vi "trial code new pid.vi"() -> ()   [LabVIEW 2025]
uses:
  <vilib>/Instr/_visa.llb/VISA Configure Serial Port (Instr).vi
  <vilib>/addons/control/pid/NI_PID_pid.lvlib
  <vilib>/addons/control/pid/pid.llb/PID (DBL).vi
  <vilib>/numeric/Random Number (Range) DBL.vi
panel:
  in  "lower bound (0)":dbl
  in  "Stroke 2":dbl
  out "error out":errorcluster
  out "Stroke RAW":dbl
  out "Stroke Tare":dbl
  in  "Boolean":bool
  in  "PID SEND":bool
  in  "PID ON":bool
  in  "Stop 3":bool
  out "output Vpp":dbl
  in  "input variable":dbl=1.0
  in  "Stop 2":bool
  out "Stroke":dbl
  out "cof":dbl
  out "Friction":dbl
  out "pizo raw":dbl
  out "LVDT Peak":dbl
  out "LVDT MAX":dbl
  out "LVDT MIN":dbl
  in  "Stroke PID Gains 2":T1={"Proportional Gain (Kc)"=200.0, "Integral Time (Ti, min)"=0.02, "Derivative Time (Td, min)"=0.0}
  in  "STROKE GAIN :":dbl=700.0 caption="Stroke Gain :"
  in  "Set Strk":dbl=1.0 caption="STROKE LENGTH" min=1.0 max=1.0 step=1.0 format="%.3f"
  in  "PID Rst":bool=TRUE
  out "Stroke PID OUT":dbl(slide)=-13.483146067415703 scale=-600.0..600.0
  out "stop cmd":bool
  out "st gain":string="0000"
  out "PID Out":u8(slide) scale=0.0..4095.0
  out "start en":bool=TRUE
  in  "command":string
  in  "Stop":bool
  in  "Com Port 2":refnum<visa-resource-name>="COM9" caption="C2 :"
  out "Residual Uno 2":string
  out "Port 1 Error 2":errorcluster={"status"=TRUE, "code"=-1073807343, "source"="Property Node (arg 1) in VISA Configure Serial Port (Instr).vi->Winducom 2010--std ed hfrr-wo1768-V18.vi"}
  out "Uno Stroke":string
  out "Sps 4":dbl
  out "Port 1a 2":bool caption="Port 1 a"
  out "Port 2":u32(graph)
  out "Error Uno 2":errorcluster={"status"=TRUE, "code"=-1073807343, "source"="Property Node (arg 1) in VISA Configure Serial Port (Instr).vi->Winducom 2010--std ed hfrr-wo1768-V18.vi"}
  out "Port 4":bool=TRUE caption="Port 1"
  in  "Re-initialize Port1 2":bool
  out "Residual Uno":string
  out "Port 1 Error":errorcluster={"status"=TRUE, "code"=-1073807343, "source"="Property Node (arg 1) in VISA Configure Serial Port (Instr).vi->Winducom 2010--std ed hfrr-wo1768-V18.vi"}
  out "due":string
  out "Sps 3":dbl
  out "Port 1a":bool caption="Port 1 a"
  out "Port 1":u32(graph)
  out "Error Uno":errorcluster={"status"=TRUE, "code"=-1073807343, "source"="Property Node (arg 1) in VISA Configure Serial Port (Instr).vi->Winducom 2010--std ed hfrr-wo1768-V18.vi"}
  out "Port 3":bool=TRUE caption="Port 1"
  in  "Re-initialize Port1":bool
  out "FF buffer":dbl[](graph)
  in  "Com Port 1":refnum<visa-resource-name>="COM7" caption="C1 :"
  out "Test \nStatus":bool caption="Test Status"
types:
  T1 = cluster{"Proportional Gain (Kc)":dbl, "Integral Time (Ti, min)":dbl, "Derivative Time (Td, min)":dbl}
  T2 = cluster{"Read Heave and Surge":string, "Bytes at Heave Port":dbl, "Heave and Surge COM Port:":refnum<visa-resource-name>, "Com Port 2":refnum<visa-resource-name>, "Residual Due":string, "Heave COM Status 2":bool, "Heave COM Status":bool, "Port 2":bool, "Sway PPR":dbl, "Surge PPR":dbl, "Heave PPR":dbl, "Sway Pitch":dbl, "Surge Pitch":dbl, "Heave Pitch":dbl, "Sway Pulses/mm":dbl, "Surge Pulses/mm":dbl, "Heave Pulses/mm":dbl, "inner loop":dbl, "Read Heave and Surge 2":string, "String 36":string, "Write S":bool, "WriteCC1":string[], "Heave COM Loop":i32, "LastCom":string, "EXIT":bool, "Error Heave":errorcluster}
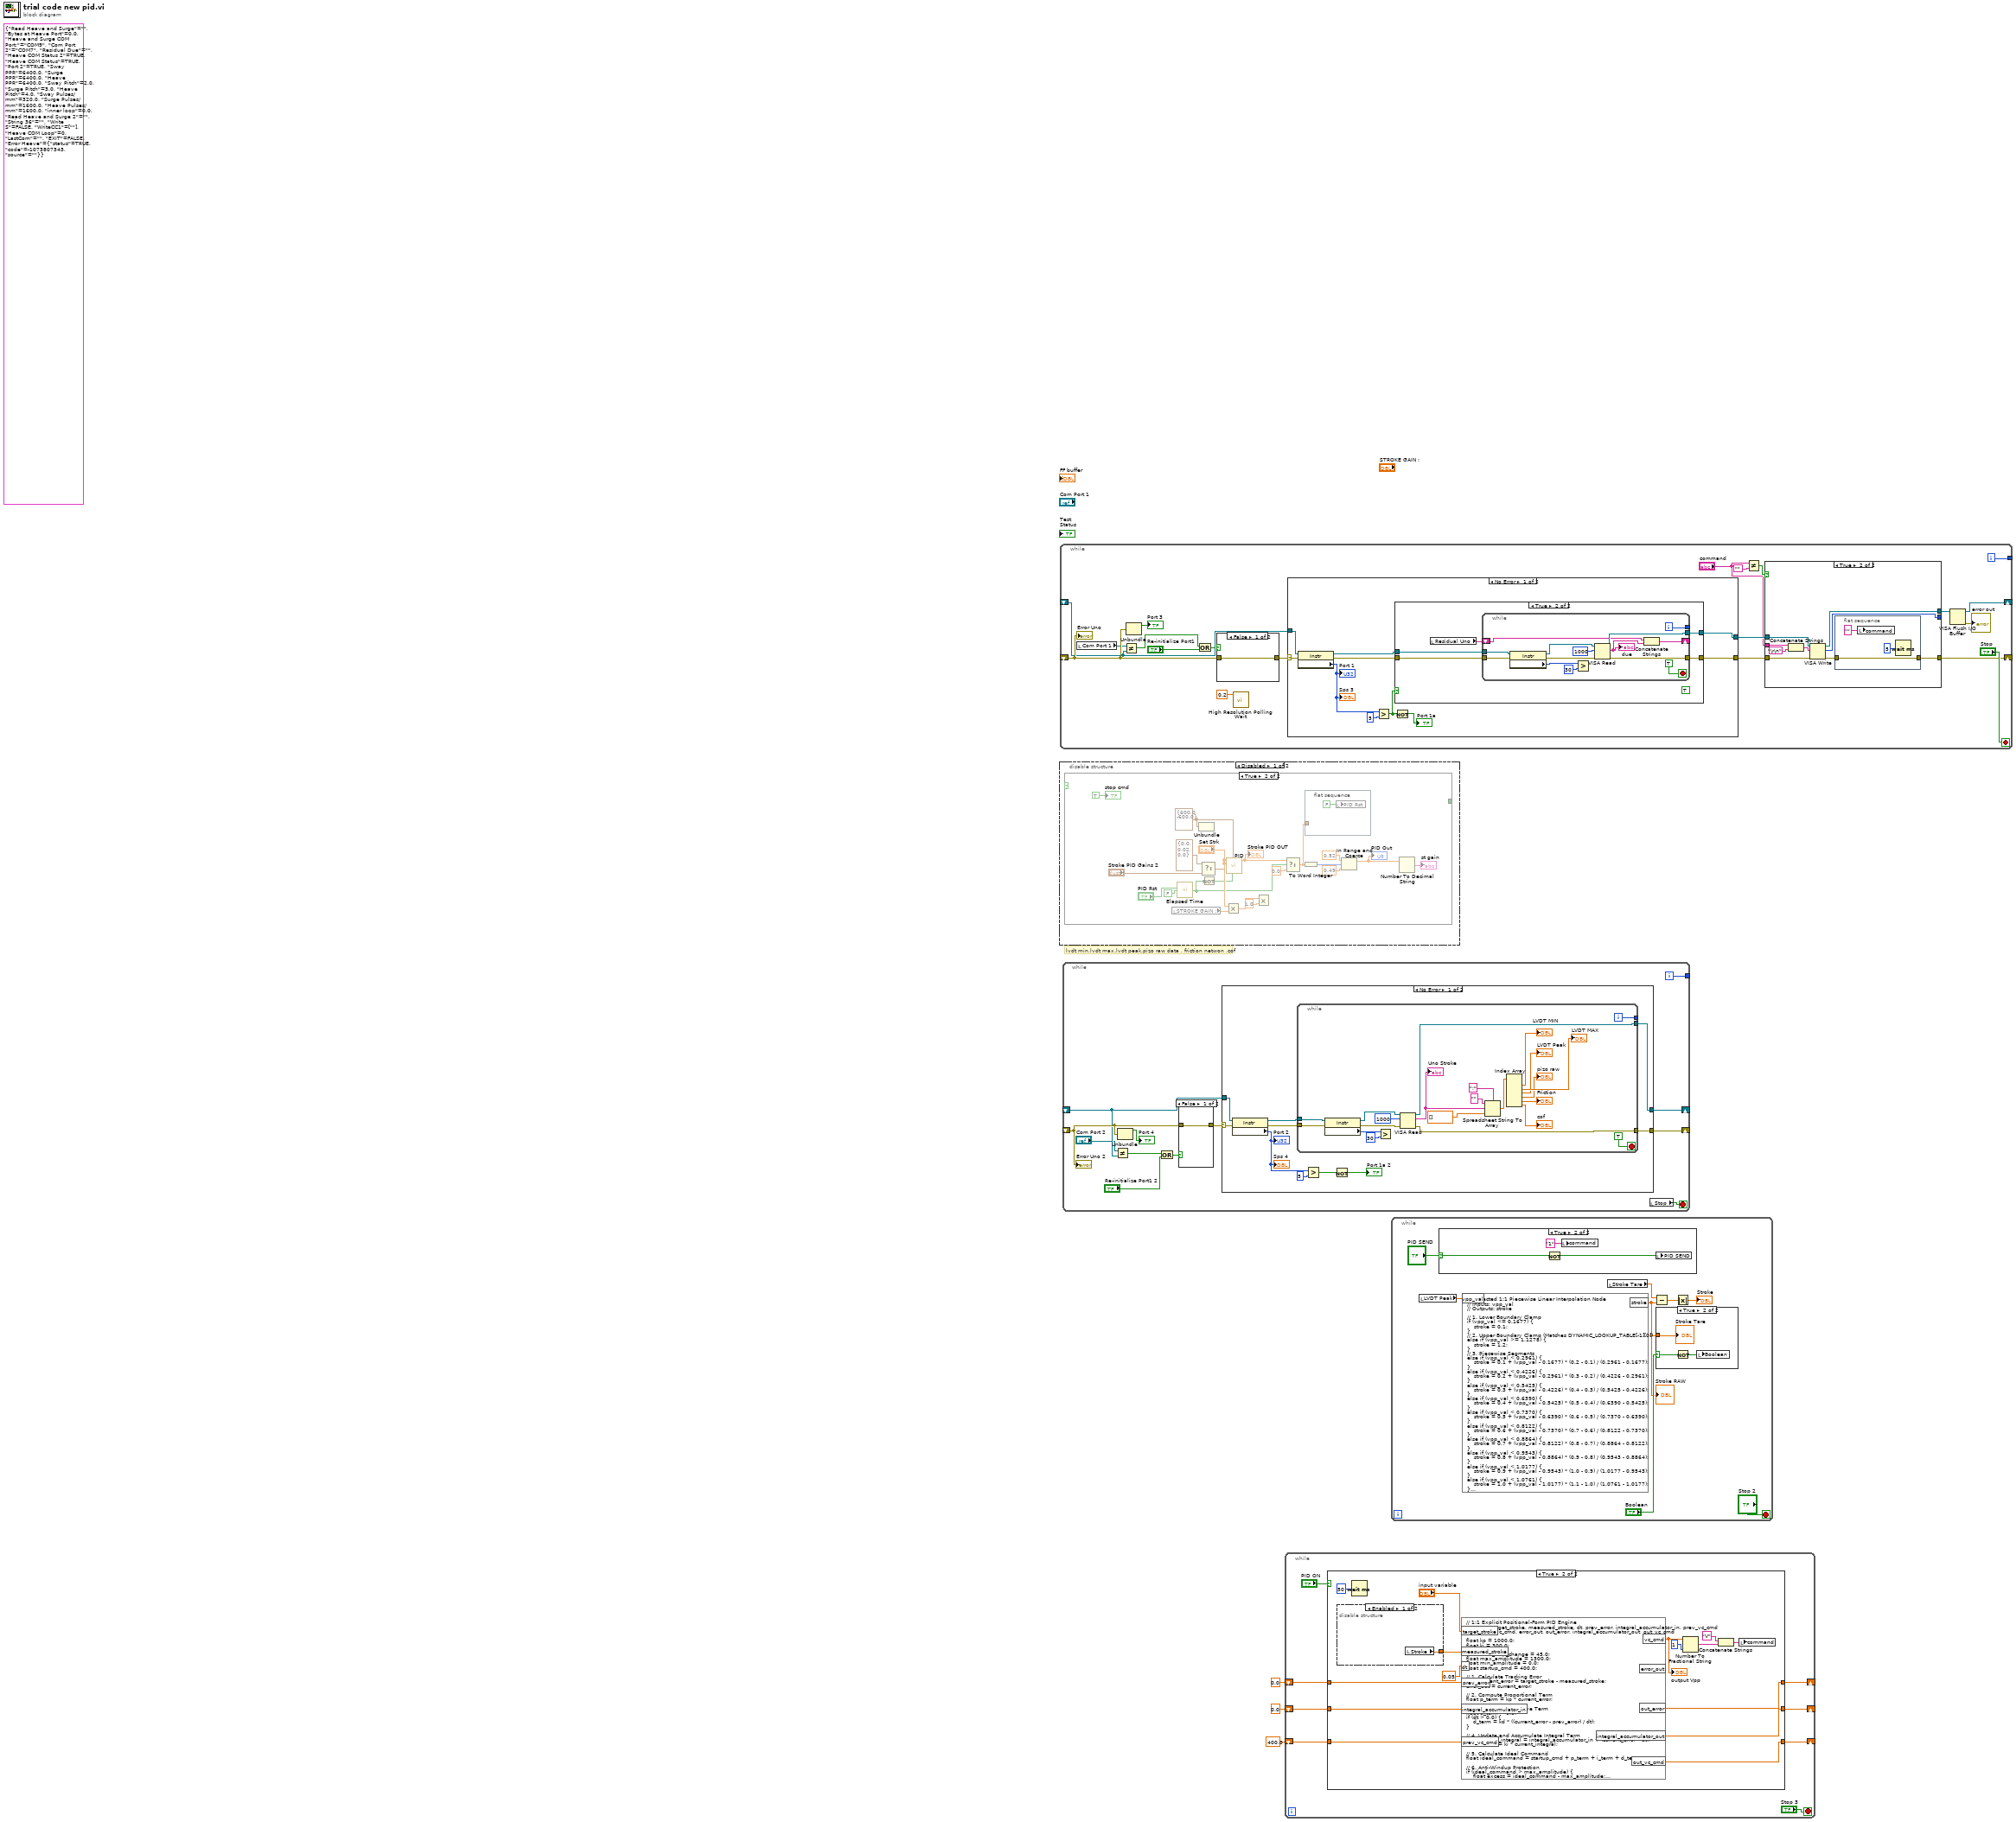
[diagram p0: block diagram]
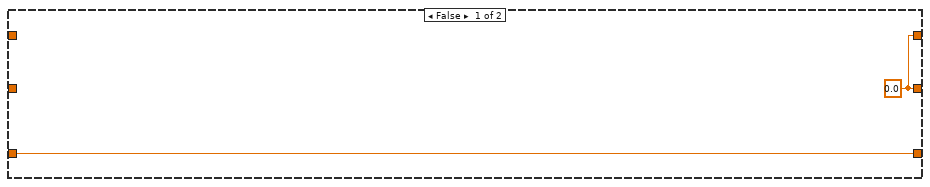
[diagram p2: hidden frame]
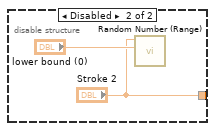
[diagram p3: hidden frame]
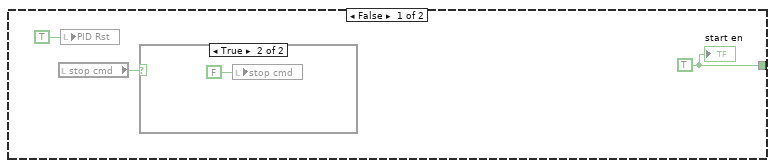
[diagram p6: hidden frame]
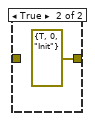
[diagram p9: hidden frame]
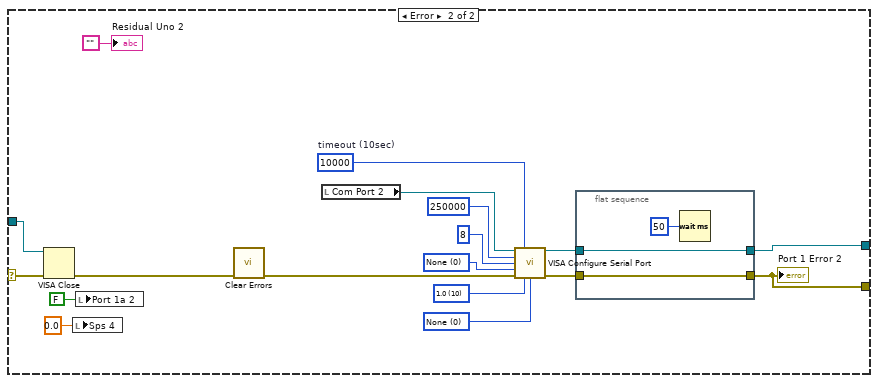
[diagram p10: hidden frame]
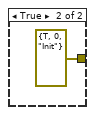
[diagram p12: hidden frame]
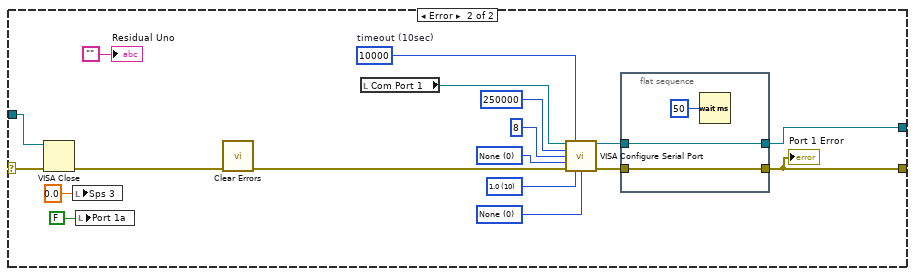
[diagram p14: hidden frame]
diagram:
  (unwired) T2 {"Read Heave and Surge"="", "Bytes at Heave Port"=0.0, "Heave and Surge COM Port:"="COM9", "Com Port 2"="COM7", "Residual Due"="", "Heave COM Status 2"=TRUE, "Heave COM Status"=TRUE, "Port 2"=TRUE, "Sway PPR"=6400.0, "Surge PPR"=6400.0, "Heave PPR"=6400.0, "Sway Pitch"=2.0, "Surge Pitch"=3.0, "Heave Pitch"=4.0, "Sway Pulses/mm"=320.0, "Surge Pulses/mm"=1600.0, "Heave Pulses/mm"=1600.0, "inner loop"=0.0, "Read Heave and Surge 2"="", "String 36"="", "Write S"=FALSE, "WriteCC1"=[""], "Heave COM Loop"=0, "LastCom"="", "EXIT"=FALSE, "Error Heave"={"status"=TRUE, "code"=-1073807343, "source"=""}}
  # "lvdt min,lvdt max,lvdt peak,pizo raw data , friction netwon ,cof"
  n1 = disable-structure shown="Disabled" {
    frame Disabled {
      n2 = case shown="True" {
        selector: _ -> [_ _]
        tunnel: [w4 _] -> _
        frame False {
          w4 = TRUE ("PID Rst")
          n3 = local read "stop cmd"() -> (w5:bool)
          n4 = local write "PID Rst"(TRUE ("PID Rst")) -> ()
          n5 = case shown="True" w5 {
            frame False {
            }
            frame True {
              n6 = local write "stop cmd"(FALSE ("stop cmd")) -> ()
            }
          }
          "start en" <- w4
        }
        frame True {
          w24 = cluster{"output high":dbl, "output low":dbl} {"output high"=600.0, "output low"=-600.0} ("output range")
          n7 = local read "STROKE GAIN :"() -> (w14:dbl)
          n8 = call "Elapsed Time"("Reset"="PID Rst", "Auto Reset"=FALSE) -> ("Time has Elapsed"=w21:bool)  [unwired: 10 in, 7 out]
          n9 = Unbundle(w24) -> ()  [unwired: 2 out]
          n10 = Select(t=T1 {"Proportional Gain (Kc)"=0.0, "Integral Time (Ti, min)"=0.02, "Derivative Time (Td, min)"=0.0} ("Stroke PID Gains"), f="Stroke PID Gains 2") -> (s? t:f=w11:T1)  [unwired: 1 in]
          n11 = Not(x=w21) -> (.not. x?=w20:bool)
          n12 = Multiply(x="Set Strk", y=w14) -> (x*y=w9:dbl)
          n13 = call-poly <vilib>:"PID.vi"("reinitialize? (F)"=w20, "output range"=w24, "PID gains"=w11, "process variable"="Set Strk", "setpoint"="Set Strk") -> ("output"=w19:dbl)  [unwired: 5 in, 1 out]
          "Stroke PID OUT" <- w19
          n14 = Multiply(x=w9, y=1.0) -> ()  [unwired: 1 out]
          n15 = Select(t=w19, s=w21, f=0.0) -> (s? t:f=w22:dbl)
          n16 = To Word Integer(number=w22) -> (16bit integer=w16:i16)
          n17 = flat-sequence {
            tunnel: w22 -> [_]
            frame #0 {
              n18 = local write "PID Rst"(FALSE ("PID Rst")) -> ()
            }
          }
          n19 = In Range and Coerce(upper limit=0.52 ("f"), x=w16, lower limit=0.49 ("f")) -> (coerced(x)=w13:dbl)  [unwired: 1 out]
          "PID Out" <- w13
          n20 = Number To Decimal String(number=w13) -> (decimal integer string=→"st gain":string)  [unwired: 1 in]
          "stop cmd" <- TRUE ("Auto Reset")
        }
      }
    }
    frame Enabled {
    }
  }
  n21 = while {
    shift-right: [w31] -> _
    shift-left: _ -> [w45]
    shift-right: [w36] -> _
    shift-left: _ -> [w47]
    tunnel: [w49] -> _
    i -> [w49]
    stop <- "Stop" stop-if-true
    n22 = local read "Com Port 1"() -> (w46:refnum<visa-resource-name>)
    n23 = Not Equal?(x=w46, y=w45) -> (x != y?=w44:bool)
    n24 = Unbundle(w47) -> ("status"=→"Port 3":bool)  [unwired: 2 out]
    n25 = Or(x=w44, y="Re-initialize Port1") -> (x .or. y?=w42:bool)
    n26 = case shown="False" w42 {
      tunnel: [w64 errorcluster {"status"=TRUE, "code"=0, "source"="Init"} ("error out")] -> w43
      tunnel: w47 -> [w64 _]
      frame False {
      }
      frame True {
      }
    }
    n27 = call <vilib>:"High Resolution Polling Wait.vi"("seconds to wait"=0.2) -> ()  [unwired: 10 in, 1 out]
    n28 = case shown="No Error" w43 {
      selector: w43 -> [w72 w102]
      tunnel: [w75 w106] -> w37
      tunnel: [w74 w99] -> w38
      tunnel: w45 -> [w73 w104]
      frame No Error {
        n29 = property class="Instr"(reference=w73, error in=w72) -> (reference out=w70:refnum<visa-resource-name>, error out=w71:errorcluster, "Serial Settings:Number of Bytes at Serial Port"=w66:u32)
        "Sps 3" <- w66
        "Port 1" <- w66
        n30 = Greater?(x=w66, y=u32 5) -> (0:w68:bool)
        n31 = Not(x=w68) -> (.not. x?=→"Port 1a":bool)
        n32 = case shown="True" w68 {
          tunnel: w70 -> [w77 w81]
          tunnel: w71 -> [w76 w79]
          tunnel: [w76 w78] -> w74
          tunnel: [w77 w82] -> w75
          frame False {
          }
          frame True {
            (unwired) TRUE ("PAUSE")
            n33 = local read "Residual Uno"() -> (w80:string)
            n34 = while {
              tunnel: [w94] -> w78
              tunnel: [w93] -> w82
              tunnel: w79 -> [w92]
              tunnel: w81 -> [w91]
              tunnel: [w89] -> _
              shift-right: [w86] -> _
              shift-left: w80 -> [w87]
              i -> [w89]
              stop <- TRUE stop-if-true
              n35 = property class="Instr"(reference=w91, error in=w92) -> (reference out=w96:refnum<visa-resource-name>, error out=w95:errorcluster, "Serial Settings:Number of Bytes at Serial Port"=w88:u32)
              n36 = Greater?(x=w88, y=u32 30) -> ()  [unwired: 1 out]
              n37 = VISA Read(VISA resource name=w96, byte count=u32 1000, error in (no error)=w95) -> (VISA resource name out=w93:refnum<visa-resource-name>, read buffer=w83:string, error out=w94:errorcluster)  [unwired: 1 out]
              "due" <- w83
              n38 = Concatenate Strings(w87, w83) -> (w86:string)
            }
          }
        }
      }
      frame Error {
        w112 = u16 0 items=["None", "XON/XOFF", "RTS/CTS", "XON/XOFF & RTS/CTS", "DTR/DSR", "XON/XOFF & DTR/DSR"] ("flow control (0:none)  2")
        w110 = u16 10 items=["1.0"=10, "1.5"=15, "2.0"=20] ("stop bits 2")
        w108 = u16 0 items=["None", "Odd", "Even", "Mark", "Space"] ("parity 2")
        w109 = u32 10000  # timeout (10sec)
        n39 = VISA Close(VISA resource name=w104, error in (no error)=w102) -> (error out=w105:errorcluster)
        n40 = local write "Sps 3"(0.0 ("Sps 4")) -> ()
        n41 = local write "Port 1a"(FALSE ("Port 1a")) -> ()
        n42 = call <vilib>:"Clear Errors.vi"("error in (no error)"=w105) -> ("error out"=w103:errorcluster)  [unwired: 5 in, 1 out]
        n43 = local read "Com Port 1"() -> (w98:refnum<visa-resource-name>)
        n44 = call-poly "VISA Configure Serial Port"("VISA resource name"=w98, "timeout (10sec)"=w109, "baud rate (9600)"=u32 250000 ("baud rate  2"), "data bits (8)"=u16 8 ("data bits  2"), "parity (0:none)"=w108, "error in (no error)"=w103, "stop bits (10: 1 bit)"=w110, "flow control (0:none)"=w112) -> ("VISA resource name out"=w113:refnum<visa-resource-name>, "error out"=w114:errorcluster)  [unwired: 6 in]
        n45 = flat-sequence {
          tunnel: w113 -> [w116]
          tunnel: w114 -> [w115]
          tunnel: [w116] -> w106
          tunnel: [w115] -> w99
          frame #0 {
            n46 = Wait (ms)(milliseconds to wait=u32 50) -> ()  [unwired: 1 out]
          }
        }
        "Residual Uno" <- ""
        "Port 1 Error" <- w99
      }
    }
    n47 = Not Equal?(x="command", y="") -> (x != y?=w33:bool)
    n48 = case shown="True" w33 {
      tunnel: w37 -> [w51 w56]
      tunnel: [w51 w60] -> w35
      tunnel: w38 -> [w50 w55]
      tunnel: [w50 w58] -> w36
      tunnel: "command" -> [_ w54]
      tunnel: [_ w57] -> _
      frame False {
        # "DATA  WRITE LOOP"
      }
      frame True {
        n49 = Concatenate Strings(w54, "\r\n") -> (w53:string)
        n50 = VISA Write(VISA resource name=w56, write buffer=w53, error in (no error)=w55) -> (VISA resource name out=w60:refnum<visa-resource-name>, return count=w57:u32, error out=w59:errorcluster)
        n51 = flat-sequence {
          tunnel: w59 -> [w62]
          tunnel: [w62] -> w58
          frame #0 {
            n52 = local write "command"("" ("command")) -> ()
            n53 = Wait (ms)(milliseconds to wait=u32 5) -> ()  [unwired: 1 out]
          }
        }
      }
    }
    n54 = VISA Flush I/O Buffer(VISA resource name=w35) -> (VISA resource name out=w31:refnum<visa-resource-name>, error out=→"error out":errorcluster)  [unwired: 2 in]
    "Error Uno" <- w47
  }
  n55 = while {
    shift-right: [w129] -> _
    shift-left: _ -> [w124]
    shift-right: [w128] -> _
    shift-left: _ -> [w125]
    tunnel: [w127] -> _
    i -> [w127]
    stop <- w118 stop-if-true
    n56 = Not Equal?(x="Com Port 2", y=w124) -> (x != y?=w123:bool)
    n57 = Unbundle(w125) -> ("status"=→"Port 4":bool)  [unwired: 2 out]
    n58 = Or(x=w123, y="Re-initialize Port1 2") -> (x .or. y?=w121:bool)
    n59 = case shown="False" w121 {
      tunnel: [w130 errorcluster {"status"=TRUE, "code"=0, "source"="Init"} ("error out")] -> w122
      tunnel: w125 -> [w130 _]
      frame False {
      }
      frame True {
      }
    }
    n60 = case shown="No Error" w122 {
      selector: w122 -> [w138 w169]
      tunnel: [w141 w173] -> w129
      tunnel: [w140 w166] -> w128
      tunnel: w124 -> [w139 w171]
      frame No Error {
        n61 = property class="Instr"(reference=w139, error in=w138) -> (reference out=w136:refnum<visa-resource-name>, error out=w137:errorcluster, "Serial Settings:Number of Bytes at Serial Port"=w132:u32)
        "Sps 4" <- w132
        "Port 2" <- w132
        n62 = while {
          tunnel: [w161] -> w140
          tunnel: [w160] -> w141
          tunnel: w137 -> [w159]
          tunnel: w136 -> [w158]
          tunnel: [w156] -> _
          i -> [w156]
          stop <- TRUE stop-if-true
          n63 = property class="Instr"(reference=w158, error in=w159) -> (reference out=w163:refnum<visa-resource-name>, error out=w162:errorcluster, "Serial Settings:Number of Bytes at Serial Port"=w155:u32)
          n64 = Greater?(x=w155, y=u32 30) -> ()  [unwired: 1 out]
          n65 = VISA Read(VISA resource name=w163, byte count=u32 1000, error in (no error)=w162) -> (VISA resource name out=w160:refnum<visa-resource-name>, read buffer=w152:string, error out=w161:errorcluster)  [unwired: 1 out]
          "Uno Stroke" <- w152
          n66 = Spreadsheet String To Array(delimiter (Tab)=";", format string="", spreadsheet string=w152, array type (2D Dbl)=dbl[] []) -> (array=w149:dbl[])
          n67 = Index Array(array=w149) -> (element #1=→"LVDT MIN":dbl, element #2=→"LVDT MAX":dbl, element #3=→"LVDT Peak":dbl, element #4=→"pizo raw":dbl, element #5=→"Friction":dbl, element #6=→"cof":dbl)  [unwired: 6 in]
        }
        n68 = Greater?(x=w132, y=u32 5) -> (0:w134:bool)
        n69 = Not(x=w134) -> (.not. x?=→"Port 1a 2":bool)
      }
      frame Error {
        w179 = u16 0 items=["None", "XON/XOFF", "RTS/CTS", "XON/XOFF & RTS/CTS", "DTR/DSR", "XON/XOFF & DTR/DSR"] ("flow control (0:none)  2")
        w177 = u16 10 items=["1.0"=10, "1.5"=15, "2.0"=20] ("stop bits 2")
        w175 = u16 0 items=["None", "Odd", "Even", "Mark", "Space"] ("parity 2")
        w176 = u32 10000  # timeout (10sec)
        n70 = VISA Close(VISA resource name=w171, error in (no error)=w169) -> (error out=w172:errorcluster)
        n71 = local write "Sps 4"(0.0 ("Sps 4")) -> ()
        n72 = local write "Port 1a 2"(FALSE ("Port 1a")) -> ()
        n73 = call <vilib>:"Clear Errors.vi"("error in (no error)"=w172) -> ("error out"=w170:errorcluster)  [unwired: 5 in, 1 out]
        n74 = local read "Com Port 2"() -> (w164:refnum<visa-resource-name>)
        n75 = call-poly "VISA Configure Serial Port"("VISA resource name"=w164, "timeout (10sec)"=w176, "baud rate (9600)"=u32 250000 ("baud rate  2"), "data bits (8)"=u16 8 ("data bits  2"), "parity (0:none)"=w175, "error in (no error)"=w170, "stop bits (10: 1 bit)"=w177, "flow control (0:none)"=w179) -> ("VISA resource name out"=w180:refnum<visa-resource-name>, "error out"=w181:errorcluster)  [unwired: 6 in]
        n76 = flat-sequence {
          tunnel: w180 -> [w183]
          tunnel: w181 -> [w182]
          tunnel: [w183] -> w173
          tunnel: [w182] -> w166
          frame #0 {
            n77 = Wait (ms)(milliseconds to wait=u32 50) -> ()  [unwired: 1 out]
          }
        }
        "Residual Uno 2" <- ""
        "Port 1 Error 2" <- w166
      }
    }
    n78 = local read "Stop"() -> (w118:bool)
    "Error Uno 2" <- w125
  }
  n79 = while {
    shift-right: [w186] -> _
    shift-left: 0.0 -> [w189]
    shift-right: [w185] -> _
    shift-left: 0.0 -> [w188]
    shift-right: [w187] -> _
    shift-left: 400.0 ("vc_cmd") -> [w192]
    stop <- "Stop 3" stop-if-true
    n80 = case shown="True" "PID ON" {
      tunnel: w192 -> [w194 w200]
      tunnel: w189 -> [_ w198]
      tunnel: w188 -> [_ w199]
      tunnel: [w194 w197] -> w187
      tunnel: [w193 w196] -> w186
      tunnel: [w193 w195] -> w185
      frame False {
        w193 = 0.0 ("error_out")
      }
      frame True {
        n81 = disable-structure shown="Enabled" {
          disable-tunnel: [w210 "Stroke 2"] -> w208
          frame Enabled {
            n82 = local read "Stroke"() -> (w210:dbl)
          }
          frame Disabled {
            n83 = call-poly <vilib>:"Random Number (Range).vi"("lower bound (0)"="lower bound (0)", "upper bound (100)"="Stroke 2") -> ()  [unwired: 9 in, 1 out]
          }
        }
        n84 = Wait (ms)(milliseconds to wait=u32 50) -> ()  [unwired: 1 out]
        n85 = formula code="// 1:1 Explicit Positional-Form PID Engine\n// Inputs: target_stroke, measured_stroke, dt, prev_error, integral_accumulator_in, prev_vc_cmd\n// Outputs: vc_cmd, error_out, out_error, integral_accumulator_out, out_vc_cmd\n\nfloat kp = 1000.0;\nfloat ki = 300.0;\nfloat kd = 40.0;\nfloat max_step_change = 45.0;\nfloat max_amplitude = 1300.0; \nfloat min_amplitude = 0.0;\nfloat startup_cmd = 400.0;\n\n// 1. Calculate Tracking Error\nfloat current_error = target_stroke - measured_stroke;\nerror_out = current_error;\n\n// 2. Compute Proportional Term\nfloat p_term = kp * current_error;\n\n// 3. Compute Derivative Term\nfloat d_term = 0.0;\nif (dt > 0.0) {\n    d_term = kd * ((current_error - prev_error) / dt);\n}\n\n// 4. Update and Accumulate Integral Term\nfloat current_integral = integral_accumulator_in + (current_error * dt);\nfloat i_term = ki * current_integral;\n\n// 5. Calculate Ideal Command\nfloat ideal_command = startup_cmd + p_term + i_term + d_term;\n\n// 6. Anti-Windup Protection\nif (ideal_command > max_amplitude) {\n    float excess = ideal_command - max_amplitude;\n    current_integral -= excess / ki;  \n    ideal_command = max_amplitude;\n} else if (ideal_command < min_amplitude) {\n    float excess = ideal_command - min_amplitude;\n    current_integral -= excess / ki;\n    ideal_command = min_amplitude;\n}\n\n// 7. Apply Python Loop Rate Limiting\nfloat raw_adjustment = ideal_command - prev_vc_cmd;\n\nif (raw_adjustment > max_step_change) {\n    raw_adjustment = max_step_change;\n} else if (raw_adjustment < -max_step_change) {\n    raw_adjustment = -max_step_change;\n}\n\nfloat next_vc_cmd = prev_vc_cmd + raw_adjustment;\n\nif (next_vc_cmd > max_amplitude) {\n    next_vc_cmd = max_amplitude;\n} else if (next_vc_cmd < min_amplitude) {\n    next_vc_cmd = min_amplitude;\n}\n\n// 8. Map to Outputs / Shift Registers\nvc_cmd = next_vc_cmd;\nout_error = current_error;                  \nintegral_accumulator_out = current_integral; \nout_vc_cmd = next_vc_cmd;"("target_stroke"="input variable", "measured_stroke"=w208, "dt"=0.05 ("input variable"), "integral_accumulator_in"=w198, "prev_error"=w199, "prev_vc_cmd"=w200) -> ("vc_cmd"=w205:dbl, "out_error"=w195:dbl, "integral_accumulator_out"=w196:dbl, "out_vc_cmd"=w197:dbl)  [unwired: 1 out]
        "output Vpp" <- w205
        n86 = Number To Fractional String(number=w205, precision (6)=i16 1) -> (F-format string=w203:string)  [unwired: 2 in]
        n87 = Concatenate Strings("V" ("string"), w203) -> (w201:string)
        n88 = local write "command"(w201) -> ()
      }
    }
  }
  n89 = while {
    stop <- "Stop 2" stop-if-true
    n90 = local read "LVDT Peak"() -> (w220:dbl)
    n91 = case shown="True" "PID SEND" {
      selector: "PID SEND" -> [_ w226]
      frame False {
      }
      frame True {
        n92 = Not(x=w226) -> (.not. x?=w225:bool)
        n93 = local write "command"("1" ("command")) -> ()
        n94 = local write "PID SEND"(w225) -> ()
      }
    }
    n95 = formula code="// Corrected 1:1 Piecewise Linear Interpolation Node\n// Inputs: vpp_val\n// Outputs: stroke\n\n// 1. Lower Boundary Clamp\nif (vpp_val <= 0.1677) {\n    stroke = 0.1;\n}\n// 2. Upper Boundary Clamp (Matches DYNAMIC_LOOKUP_TABLE[-1][0])\nelse if (vpp_val >= 1.1278) {\n    stroke = 1.2;\n}\n// 3. Piecewise Segments \nelse if (vpp_val < 0.2961) {\n    stroke = 0.1 + (vpp_val - 0.1677) * (0.2 - 0.1) / (0.2961 - 0.1677);\n}\nelse if (vpp_val < 0.4226) {\n    stroke = 0.2 + (vpp_val - 0.2961) * (0.3 - 0.2) / (0.4226 - 0.2961);\n}\nelse if (vpp_val < 0.5425) {\n    stroke = 0.3 + (vpp_val - 0.4226) * (0.4 - 0.3) / (0.5425 - 0.4226);\n}\nelse if (vpp_val < 0.6390) {\n    stroke = 0.4 + (vpp_val - 0.5425) * (0.5 - 0.4) / (0.6390 - 0.5425);\n}\nelse if (vpp_val < 0.7370) {\n    stroke = 0.5 + (vpp_val - 0.6390) * (0.6 - 0.5) / (0.7370 - 0.6390);\n}\nelse if (vpp_val < 0.8122) {\n    stroke = 0.6 + (vpp_val - 0.7370) * (0.7 - 0.6) / (0.8122 - 0.7370);\n}\nelse if (vpp_val < 0.8864) {\n    stroke = 0.7 + (vpp_val - 0.8122) * (0.8 - 0.7) / (0.8864 - 0.8122);\n}\nelse if (vpp_val < 0.9543) {\n    stroke = 0.8 + (vpp_val - 0.8864) * (0.9 - 0.8) / (0.9543 - 0.8864);\n}\nelse if (vpp_val < 1.0177) {\n    stroke = 0.9 + (vpp_val - 0.9543) * (1.0 - 0.9) / (1.0177 - 0.9543);\n}\nelse if (vpp_val < 1.0761) {\n    stroke = 1.0 + (vpp_val - 1.0177) * (1.1 - 1.0) / (1.0761 - 1.0177);\n}\nelse {\n    stroke = 1.1 + (vpp_val - 1.0761) * (1.2 - 1.1) / (1.1278 - 1.0761);\n}"("vpp_val"=w220) -> ("stroke"=w215:dbl)
    "Stroke RAW" <- w215
    n96 = local read "Stroke Tare"() -> (w216:dbl)
    n97 = Subtract(x=w216, y=w215) -> (x-y=w214:dbl)
    n98 = case shown="True" "Boolean" {
      selector: "Boolean" -> [_ w223]
      tunnel: w215 -> [_ w221]
      frame False {
      }
      frame True {
        n99 = Not(x=w223) -> (.not. x?=w222:bool)
        n100 = local write "Boolean"(w222) -> ()
        "Stroke Tare" <- w221
      }
    }
    n101 = Absolute Value(x=w214) -> (abs(x)=→"Stroke":dbl)
  }
